vi "Initialize_Control.vi"(0 "ERD Loop":refnum<queue>, 2 "GEA2":refnum<queue>, 5 "Receive Loop":T2, 7 "UI Loop Error":T1, 9 "Cont Send":refnum<queue>, 11 "Error In":errorcluster, 13 "DAQ":refnum<queue>) -> (15 "Error Out":errorcluster)   [LabVIEW 2021]
uses:
  type defs/ERD_Data_Loop_Control.ctl
  type defs/ERD_Loop_States.ctl
  Common/GExplorer Support/typedefs/GExplorer_Data_Cluster.ctl
  type defs/DAQ_States.ctl
  type defs/Ref_ReceiveLoop_Error_UserEvent.ctl
  type defs/Ref_UILoop_Error_UserEvent.ctl
  type defs/Cont_Send_States.ctl
  type defs/Error_Command.ctl
  type defs/ERD_Loop_Control_Command.ctl
  type defs/DAQ_Control_Command.ctl
  type defs/GEA2_Control_Command.ctl
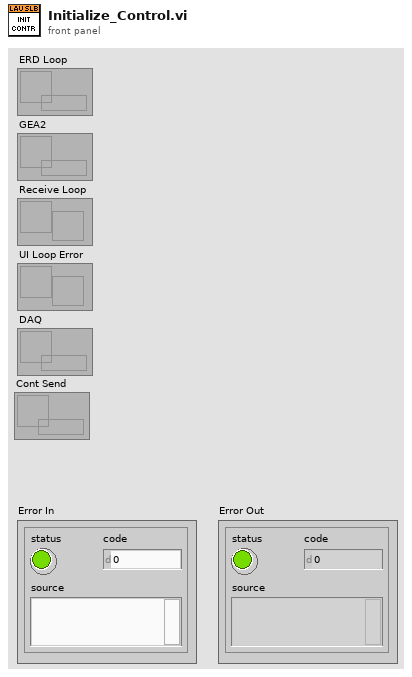
[diagram p1: front panel]
types:
  T1 = typedef "Ref_UILoop_Error_UserEvent.ctl" = refnum<user-event>
  T2 = typedef "Ref_ReceiveLoop_Error_UserEvent.ctl" = refnum<user-event>
  T3 = typedef "GEA2_Control_Command.ctl" = enum16{"Initialize", "Shutdown"}
  T4 = typedef "DAQ_Control_Command.ctl" = enum16{"Initialize", "Shutdown", "Exit"}
  T5 = typedef "ERD_Loop_Control_Command.ctl" = enum16{"Initialize", "Shutdown"}
  T6 = typedef "Error_Command.ctl" = enum16{"Initialize", "Handle Errors", "Report Errors"}
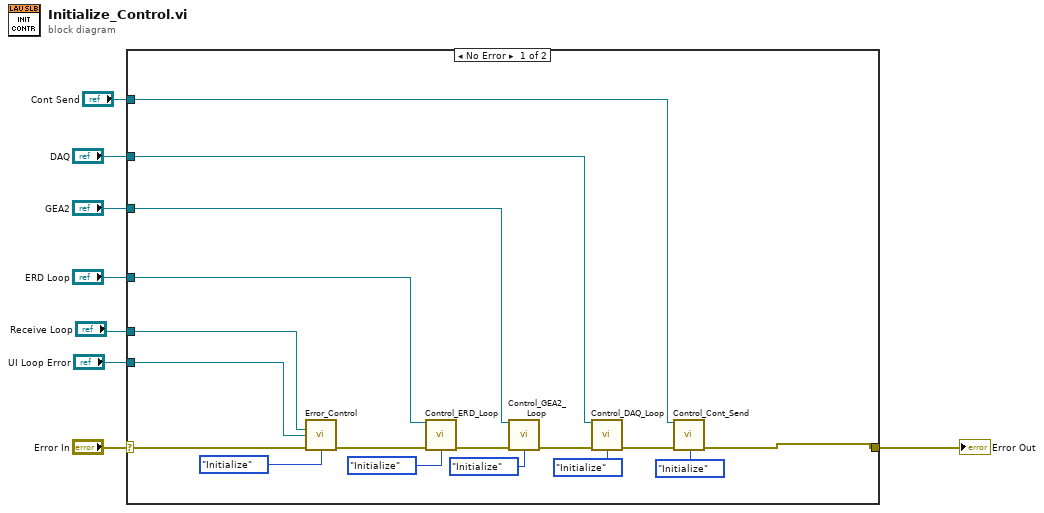
[diagram p0: block diagram]
diagram:
  n1 = case shown="No Error" "Error In" {
    selector: "Error In" -> [w19 w26]
    tunnel: [w9 w26] -> w7
    tunnel: "Receive Loop" -> [w13 _]
    tunnel: "ERD Loop" -> [w18 _]
    tunnel: "GEA2" -> [w17 _]
    tunnel: "DAQ" -> [w15 _]
    tunnel: "UI Loop Error" -> [w14 _]
    tunnel: "Cont Send" -> [w10 _]
    frame No Error {
      n2 = call "Error_Control.vi"("Command (Handle Errors)"=Error_Command."Initialize", "Receive Loop"=w13, "UI Loop Error"=w14, "Error In"=w19) -> ("Error Out"=w20:errorcluster)  [unwired: 11 in]
      n3 = call "Control_ERD_Loop.vi"("ERD Loop"=w18, "Command (ERD Loop Control)"=ERD_Loop_Control_Command."Initialize", "Error In"=w20) -> ("Error Out"=w23:errorcluster)  [unwired: 12 in]
      n4 = call "Control_GEA2_Loop.vi"("GEA2"=w17, "Command (ERD Loop Control)"=GEA2_Control_Command."Initialize", "Error In"=w23) -> ("Error Out"=w21:errorcluster)  [unwired: 12 in]
      n5 = call "Control_DAQ_Loop.vi"("DAQ"=w15, "Command (DAQ Control)"=DAQ_Control_Command."Initialize", "Error In"=w21) -> ("Error Out"=w12:errorcluster)  [unwired: 12 in]
      n6 = call "Control_Cont_Send.vi"("Cont Send"=w10, "Command (ERD Loop Control)"=GEA2_Control_Command."Initialize", "Error In"=w12) -> ("Error Out"=w9:errorcluster)  [unwired: 12 in]
    }
    frame Error {
    }
  }
  "Error Out" <- w7
